vi "V2 - Client.vi"() -> ()   [LabVIEW 2024]
panel:
  in  "Server Closed":string="The server VI closed the connection."
  in  "Stop":bool
  out "Waveform Graph":dbl[](graph)
  out "*(type *) &x":dbl[](array[numeric])
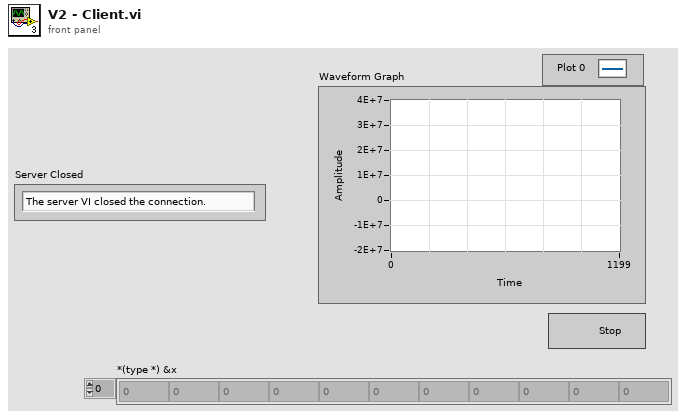
[diagram p1: front panel]
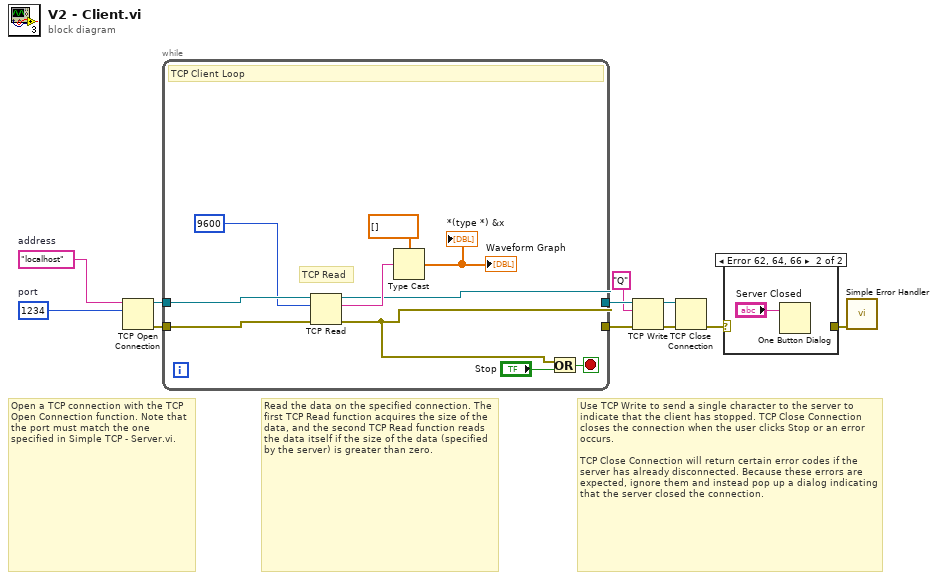
[diagram p0: block diagram]
diagram:
  w1 = u16 1234  # port
  w2 = "localhost"  # address
  # "Use TCP Write to send a single character to the server to indicate that the client has stopped. TCP Close Connection closes the connection when the user clicks Stop or an error occurs.\n\nTCP Close Connection will return certain error codes if the server has already disconnected. Because these errors are expected, ignore them and instead pop up a dialog indicating that the server closed the connection."
  # "Read the data on the specified connection. The first TCP Read function acquires the size of the data, and the second TCP Read function reads the data itself if the size of the data (specified by the server) is greater than zero."
  # "Open a TCP connection with the TCP Open Connection function. Note that the port must match the one specified in Simple TCP - Server.vi."
  n1 = TCP Open Connection(address=w2, remote port or service name=w1) -> (connection ID=w11:refnum<k5>, error out=w10:errorcluster)  [unwired: 3 in]
  n2 = while {
    tunnel: w10 -> [w13]
    tunnel: w11 -> [w14]
    tunnel: [w15] -> w8
    tunnel: [w16] -> w6
    stop <- w20 stop-if-true
    # "TCP Read"
    # "TCP Client Loop"
    n3 = TCP Read(connection ID=w14, bytes to read=9600, error in (no error)=w13) -> (connection ID out=w15:refnum<k5>, data out=w19:string, error out=w16:errorcluster)  [unwired: 2 in]
    n4 = Type Cast(type=dbl[] [] ("chart"), x=w19) -> (*(type *) &x=→"Waveform Graph" →"*(type *) &x":dbl[])
    n5 = Or(x=w16, y="Stop") -> (x .or. y?=w20:bool)
  }
  n6 = TCP Write(connection ID=w8, data in="Q", error in (no error)=w6) -> (connection ID out=w9:refnum<k5>, error out=w7:errorcluster)  [unwired: 2 out]
  n7 = TCP Close Connection(connection ID=w9, error in (no error)=w7) -> (error out=w4:errorcluster)  [unwired: 1 in, 1 out]
  n8 = case shown="Error 62, 64, 66" w4 {
    selector: w4 -> [w22 _]
    tunnel: [w22 _] -> w3
    frame #0 {
    }
    frame #1 {
      n9 = One Button Dialog(message="Server Closed") -> ()  [unwired: 1 in, 1 out]
    }
  }
  n10 = call <vilib>:"Simple Error Handler.vi"("error in (no error)"=w3) -> ()  [unwired: 4 in, 5 out]
